vi "Init Tree Control.vi"(8 "Error in":errorcluster caption="Error in (no error)", 11 "TreeControl in":refnum<vi>) -> (0 "Error out":errorcluster, 3 "TreeControl out":refnum<vi>)   [LabVIEW 2018, in "VILab.lvlib"]
uses:
  VILab.lvlib
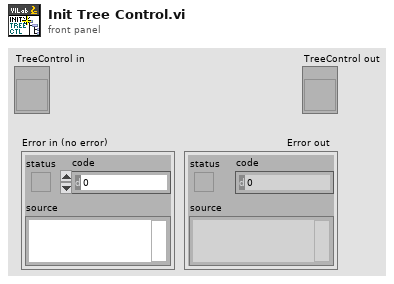
[diagram p1: front panel]
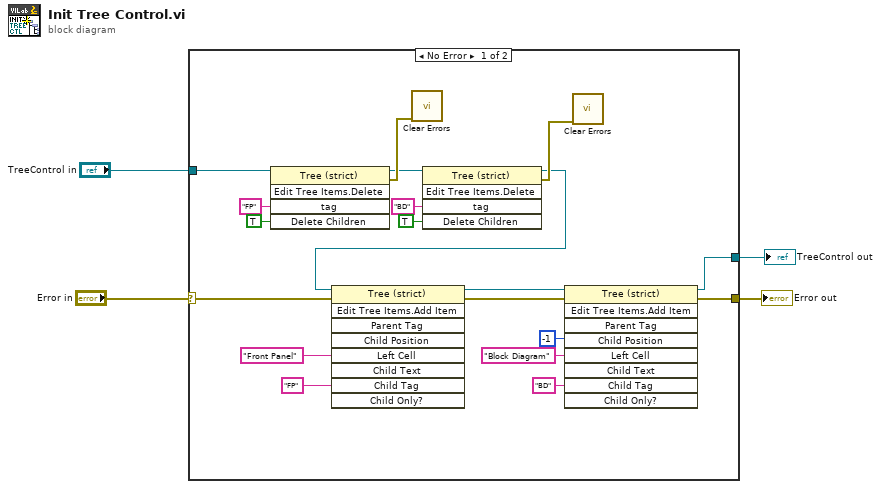
[diagram p0: block diagram]
diagram:
  n1 = case shown="No Error" "Error in" {
    selector: "Error in" -> [w8 w24]
    tunnel: "TreeControl in" -> [w9 w25]
    tunnel: [w6 w24] -> w2
    tunnel: [w5 w25] -> w1
    frame No Error {
      n2 = invoke class="Tree (strict)" method="Edit Tree Items.Delete"(reference=w9, "tag"="FP" ("Tag"), "Delete Children"=TRUE ("Delete Children?")) -> (reference out=w12:refnum<vi>, error out=w22:errorcluster)  [unwired: 2 in, 3 out]
      n3 = call <vilib>:"Clear Errors.vi"("error in (no error)"=w22) -> ()  [unwired: 5 in, 2 out]
      n4 = invoke class="Tree (strict)" method="Edit Tree Items.Delete"(reference=w12, "tag"="BD" ("Tag"), "Delete Children"=TRUE ("Delete Children?")) -> (reference out=w17:refnum<vi>, error out=w21:errorcluster)  [unwired: 2 in, 3 out]
      n5 = invoke class="Tree (strict)" method="Edit Tree Items.Add Item"(reference=w17, error in=w8, "Left Cell"="Front Panel" ("Left Cell String"), "Child Tag"="FP") -> (reference out=w18:refnum<vi>, error out=w7:errorcluster)  [unwired: 5 in, 7 out]
      n6 = invoke class="Tree (strict)" method="Edit Tree Items.Add Item"(reference=w18, error in=w7, "Child Position"=-1, "Left Cell"="Block Diagram" ("Left Cell String"), "Child Tag"="BD") -> (reference out=w5:refnum<vi>, error out=w6:errorcluster)  [unwired: 4 in, 7 out]
      n7 = call <vilib>:"Clear Errors.vi"("error in (no error)"=w21) -> ()  [unwired: 5 in, 2 out]
    }
    frame Error {
    }
  }
  "Error out" <- w2
  "TreeControl out" <- w1
